vi "ConfigDa.vi"(0 "Pump_1AI_1DO_2DI in":refnum<class "Valve_2DO_2DI.lvclass">, 11 "error in (no error)":errorcluster) -> (4 "Pump_1AI_1DO_2DI out":refnum<class "Valve_2DO_2DI.lvclass">, 15 "error out":errorcluster)   [LabVIEW 2019, in "Valve_2DO_2DI.lvclass"]
uses:
  Valve_2DO_2DI.lvclass
  D:/GIT H4000/H4000/src/Proccess_class/Proccess.lvclass
  Proccess_class/TAGs.ctl
  TypeDef/bool_setting.ctl
  DA_class/DA.lvclass
  Proccess_class/Proccess.lvclass/Proccess.ctl
  Valve_2DO_2DI.lvclass/Valve_2DO_2DI.ctl
  Proccess_class/Proccess.lvclass
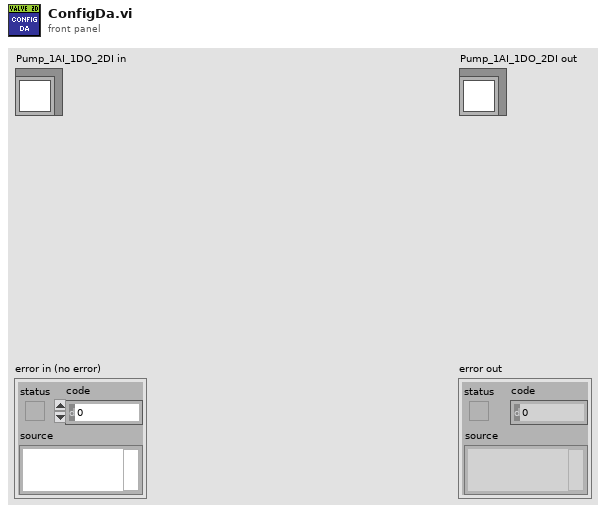
[diagram p1: front panel]
types:
  T1 = typedef "bool_setting.ctl" = cluster{"TON_ms":u32, "TOFF_ms":u32}
  T2 = typedef "Proccess.lvclass/TAGs.ctl" = cluster{"TAG":string, "PTAG":string, "DESC":string}
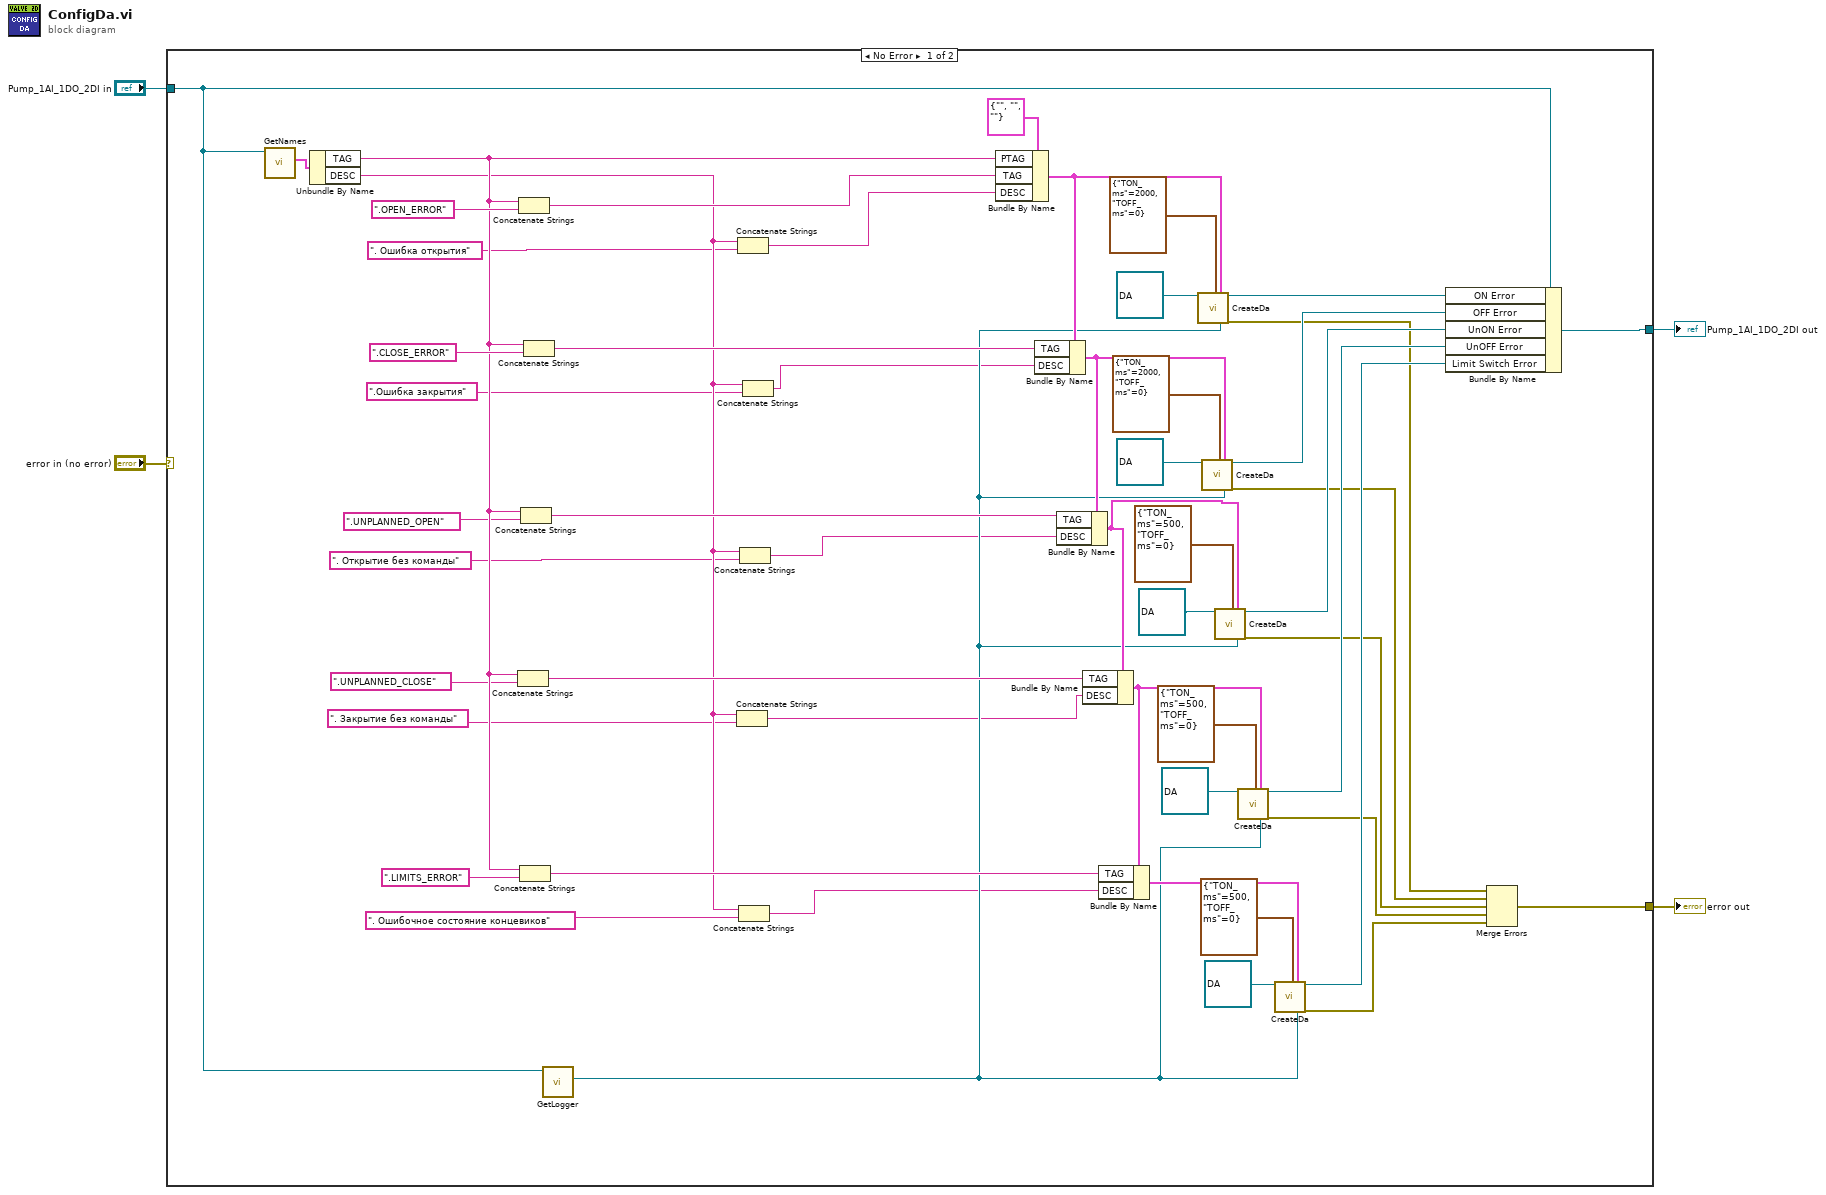
[diagram p0: block diagram]
diagram:
  n1 = case shown="No Error" "error in (no error)" {
    selector: "error in (no error)" -> [_ w59]
    tunnel: [w18 w59] -> w1
    tunnel: [w57 w58] -> w3
    tunnel: "Pump_1AI_1DO_2DI in" -> [w56 w58]
    frame No Error {
      n2 = call "GetNames.vi"("Proccess in"=w56) -> ("Tags"=w53:T2)  [unwired: 10 in]
      n3 = Unbundle By Name(w53) -> ("TAG"=w47:string, "DESC"=w17:string)
      n4 = Concatenate Strings(w47, ".UNPLANNED_CLOSE" ("string")) -> (w33:string)
      n5 = Concatenate Strings(w47, ".OPEN_ERROR" ("string")) -> (w50:string)
      n6 = Concatenate Strings(w47, ".LIMITS_ERROR" ("string")) -> (w26:string)
      n7 = Concatenate Strings(w47, ".UNPLANNED_OPEN" ("string")) -> (w38:string)
      n8 = Concatenate Strings(w47, ".CLOSE_ERROR" ("string")) -> (w42:string)
      n9 = call "GetLogger.vi"("Proccess in"=w56) -> ("Logger"=w24:refnum<class "Logger.lvclass">)  [unwired: 10 in]
      n10 = Concatenate Strings(w17, ". Закрытие без команды" ("string")) -> (w13:string)
      n11 = Concatenate Strings(w17, ". Ошибка открытия" ("string")) -> (w16:string)
      n12 = Concatenate Strings(w17, ". Ошибочное состояние концевиков" ("string")) -> (w12:string)
      n13 = Concatenate Strings(w17, ". Открытие без команды" ("string")) -> (w14:string)
      n14 = Concatenate Strings(w17, ".Ошибка закрытия" ("string")) -> (w15:string)
      n15 = Bundle By Name(cluster=T2 {"TAG"="", "PTAG"="", "DESC"=""} ("Tags"), "PTAG"=w47, "TAG"=w50, "DESC"=w16) -> (w43:T2)
      n16 = Bundle By Name(cluster=w43, "TAG"=w42, "DESC"=w15) -> (w37:T2)
      n17 = Bundle By Name(cluster=w37, "TAG"=w38, "DESC"=w14) -> (w32:T2)
      n18 = Bundle By Name(cluster=w32, "TAG"=w33, "DESC"=w13) -> (w27:T2)
      n19 = Bundle By Name(cluster=w27, "TAG"=w26, "DESC"=w12) -> (w30:T2)
      n20 = call "CreateDa.vi"("Sig_DA in"=refnum<class "DA.lvclass"> refnum ("Sig_DA"), "bool_setting"=T1 {"TON_ms"=2000, "TOFF_ms"=0}, "Tags"=w43, "Logger"=w24) -> ("Sig_DA out"=w45:refnum<class "DA.lvclass">, "error out"=w19:errorcluster)  [unwired: 14 in]
      n21 = call "CreateDa.vi"("Sig_DA in"=refnum<class "DA.lvclass"> refnum ("Sig_DA"), "bool_setting"=T1 {"TON_ms"=2000, "TOFF_ms"=0}, "Tags"=w37, "Logger"=w24) -> ("Sig_DA out"=w44:refnum<class "DA.lvclass">, "error out"=w20:errorcluster)  [unwired: 14 in]
      n22 = call "CreateDa.vi"("Sig_DA in"=refnum<class "DA.lvclass"> refnum ("Sig_DA"), "bool_setting"=T1 {"TON_ms"=500, "TOFF_ms"=0}, "Tags"=w32, "Logger"=w24) -> ("Sig_DA out"=w36:refnum<class "DA.lvclass">, "error out"=w21:errorcluster)  [unwired: 14 in]
      n23 = call "CreateDa.vi"("Sig_DA in"=refnum<class "DA.lvclass"> refnum ("Sig_DA"), "bool_setting"=T1 {"TON_ms"=500, "TOFF_ms"=0}, "Tags"=w27, "Logger"=w24) -> ("Sig_DA out"=w31:refnum<class "DA.lvclass">, "error out"=w22:errorcluster)  [unwired: 14 in]
      n24 = call "CreateDa.vi"("Sig_DA in"=refnum<class "DA.lvclass"> refnum ("Sig_DA"), "bool_setting"=T1 {"TON_ms"=500, "TOFF_ms"=0}, "Tags"=w30, "Logger"=w24) -> ("Sig_DA out"=w25:refnum<class "DA.lvclass">, "error out"=w23:errorcluster)  [unwired: 14 in]
      n25 = Bundle By Name(cluster=w56, "ON Error"=w45, "OFF Error"=w44, "UnON Error"=w36, "UnOFF Error"=w31, "Limit Switch Error"=w25) -> (w57:refnum<class "Valve_2DO_2DI.lvclass">)
      n26 = Merge Errors(w19, w20, w21, w22, w23) -> (w18:errorcluster)
    }
    frame Error {
    }
  }
  "error out" <- w1
  "Pump_1AI_1DO_2DI out" <- w3
